vi "set_settings_cluster.vi"(8 "error in (no error)":errorcluster, 10 "settings cluster in":variant, 11 "ScanModeMG091111IntrinsicImaging in":refnum<class "ImagingModeMG091111IntrinsicImaging.lvclass">) -> (0 "error out":errorcluster, 3 "ScanModeMG091111IntrinsicImaging out":refnum<class "ImagingModeMG091111IntrinsicImaging.lvclass">)   [LabVIEW 2010, in "ImagingModeMG091111IntrinsicImaging.lvclass"]
uses:
  ImagingModeMG091111IntrinsicImaging.lvclass
  ImagingModeMG091111IntrinsicImaging.lvclass/ImagingModeMG091111IntrinsicImaging.ctl
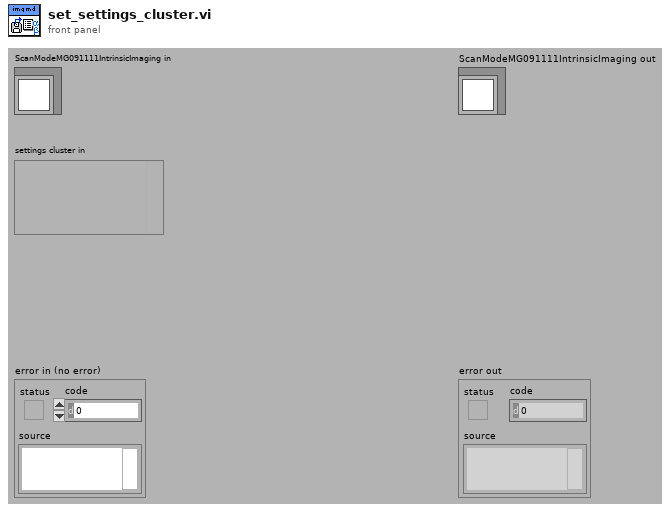
[diagram p1: front panel]
types:
  T1 = typedef "ImagingModeMG091111IntrinsicImaging.lvclass/settings_cluster.ctl" = cluster{"SkipControl":bool, "PhaseDuration":dbl[unit], "OffsetTime":dbl[unit], "ImageWidth":i32, "ImageHeight":i32, "FrameRate":dbl[unit]}
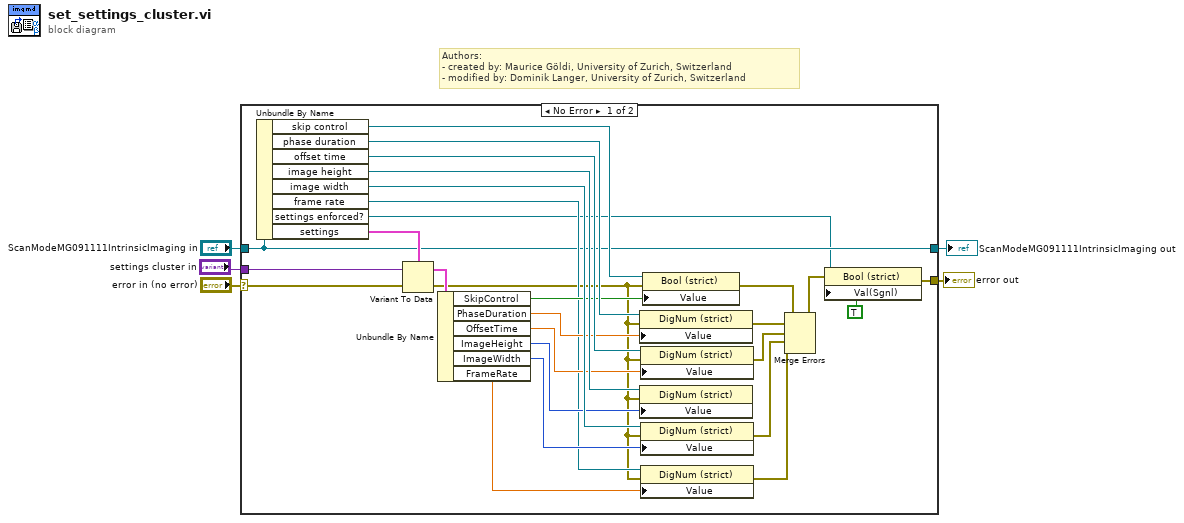
[diagram p0: block diagram]
diagram:
  # "Authors: \n- created by: Maurice Göldi, University of Zurich, Switzerland\n- modified by: Dominik Langer, University of Zurich, Switzerland"
  n1 = case shown="No Error" "error in (no error)" {
    selector: "error in (no error)" -> [w13 w34]
    tunnel: [w9 w34] -> w5
    tunnel: [w14 w33] -> w4
    tunnel: "ScanModeMG091111IntrinsicImaging in" -> [w14 w33]
    tunnel: "settings cluster in" -> [w12 _]
    frame No Error {
      n2 = Unbundle By Name(w14) -> ("skip control"=w30:refnum<vi>, "phase duration"=w29:refnum<vi>, "offset time"=w28:refnum<vi>, "image height"=w27:refnum<vi>, "image width"=w26:refnum<vi>, "frame rate"=w19:refnum<vi>, "settings enforced?"=w7:refnum<vi>, "settings"=w31:T1)
      n3 = Variant To Data(error in=w13, Variant=w12, type=w31) -> (error out=w11:errorcluster, data=w32:T1)
      n4 = Unbundle By Name(w32) -> ("SkipControl"=w25:bool, "PhaseDuration"=w24:dbl[unit], "OffsetTime"=w23:dbl[unit], "ImageHeight"=w22:i32, "ImageWidth"=w21:i32, "FrameRate"=w20:dbl[unit])
      n5 = property class="DigNum (strict)"(reference=w29, error in=w11, "Value"=w24) -> (error out=w18:errorcluster)  [unwired: 1 out]
      n6 = property class="DigNum (strict)"(reference=w27, error in=w11, "Value"=w22) -> ()  [unwired: 2 out]
      n7 = property class="DigNum (strict)"(reference=w28, error in=w11, "Value"=w23) -> (error out=w17:errorcluster)  [unwired: 1 out]
      n8 = property class="DigNum (strict)"(reference=w26, error in=w11, "Value"=w21) -> (error out=w16:errorcluster)  [unwired: 1 out]
      n9 = property class="DigNum (strict)"(reference=w19, error in=w11, "Value"=w20) -> (error out=w15:errorcluster)  [unwired: 1 out]
      n10 = property class="Bool (strict)"(reference=w30, error in=w11, "Value"=w25) -> (error out=w10:errorcluster)  [unwired: 1 out]
      n11 = Merge Errors(w10, w18, w17, w16, w15) -> (w8:errorcluster)
      n12 = property class="Bool (strict)"(reference=w7, error in=w8, "Val(Sgnl)"=TRUE ("Value (Signaling)")) -> (error out=w9:errorcluster)  [unwired: 1 out]
    }
    frame Error {
    }
  }
  "error out" <- w5
  "ScanModeMG091111IntrinsicImaging out" <- w4
